vi "006 gràfic temperatura.vi"() -> ()   [LabVIEW 2019]
panel:
  out "Waveform Chart":dbl(graph)
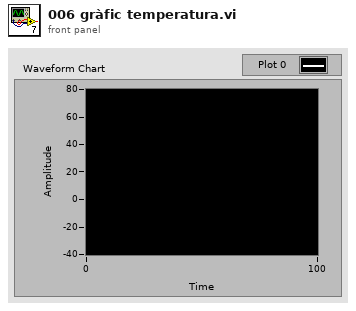
[diagram p1: front panel]
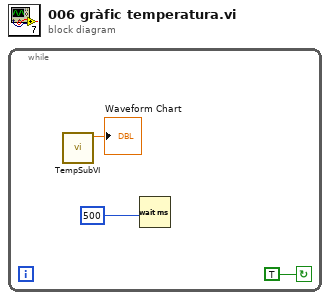
[diagram p0: block diagram]
diagram:
  n1 = while {
    stop <- TRUE continue-if-true
    n2 = call "TempSubVI.vi"() -> ("temp"=→"Waveform Chart":dbl)  [unwired: 11 in]
    n3 = Wait (ms)(milliseconds to wait=500) -> ()  [unwired: 1 out]
  }
